vi "Configure Slave Test.vi"(8 "error in (no error)":errorcluster) -> (0 "error out":errorcluster)   [LabVIEW 2015]
uses:
  Tests/Controls/Test Config.ctl
  Tests/Controls/Gas Mixture.ctl
  CAN Communication/PAS/Typedefs/ADC Gains.ctl
  Tests/Controls/Filter Sequence.ctl
  Tests/Controls/Functional Test.ctl
  CAN Communication/PAS/PAS.lvclass
panel:
  in  "Test Config":T1={"Chopper RPM"=140, "IR Power"=5, "Conc Tolerance"=0.0, "Gas Stable Time"=0, "A-D Settle"=0, "Samples"=0, "Filter Time"=0, "Gas Mixtures"=[], "Filter Sequences"=[], "Functional Test"={"Mic Test ON ADC Max"=0.0, "Mic Test ON ADC Min"=0.0, "Mic Test OFF ADC Max"=0.0, "Mic Test OFF ADC Min"=0.0, "Mic Test IC ADC Max"=0.0, "Mic Test IC ADC Min"=0.0, "IR Emitter ON ADC Max"=0.0, "IR Emitter ON ADC Min"=0.0, "IR Emitter OFF ADC Max"=0.0, "IR Emitter OFF ADC Min"=0.0}, "Initial Flow Rate"=0.0, "Max Flow Rate"=0.0} {"Gas Mixtures"."ADC Gains" items=["0"=0, "3"=3, "4"=4, "5"=5, "6"=6, "7"=7]; "Conc Tolerance" min=0.0 max=100.0 step=1.0; "IR Power" min=2 max=5 step=1; "Chopper RPM" min=140 max=1000 step=1}
  in  "Remove Filter":bool
  in  "Max Flow Rate":sgl caption="Max Flow Rate (ccm)"
  in  "Initial Flow Rate":sgl caption="Initial Flow Rate (ccm)"
  in  "Down Button":bool
  in  "Up Button":bool
  in  "Edit Gas":bool
  in  "Add Gas":bool
  in  "Remove Gas":bool
  in  "Phase Per Filter":i32(listbox)=-2
  in  "Filter Time":u16 caption="Filter Settling Time (s)"
  in  "Samples":u16
  in  "A-D Settle":u16 caption="ADC Sampling Time (ms)"
  in  "Gas Stable Time":u16 caption="Gas Stability Time (s)"
  in  "Conc Tolerance":dbl caption="Concentration Tolerance (%)" min=0.0 max=100.0 step=1.0
  in  "IR Power":u8=5 caption="IR Power (W)" min=2 max=5 step=1
  in  "Chopper RPM":u16=140 caption="Chopper Frequency (RPM)" min=140 max=1000 step=1
  in  "Gas Mixtures":i32(listbox)=-2
  out "Cancelled?":bool
  in  "Cancel Button":bool
  in  "OK Button":bool
  out "Test Sequence":i32(listbox)=-2
  # "Configure Test"
  # "Hover over the controls\nto learn more about \nthe configuraton settings"
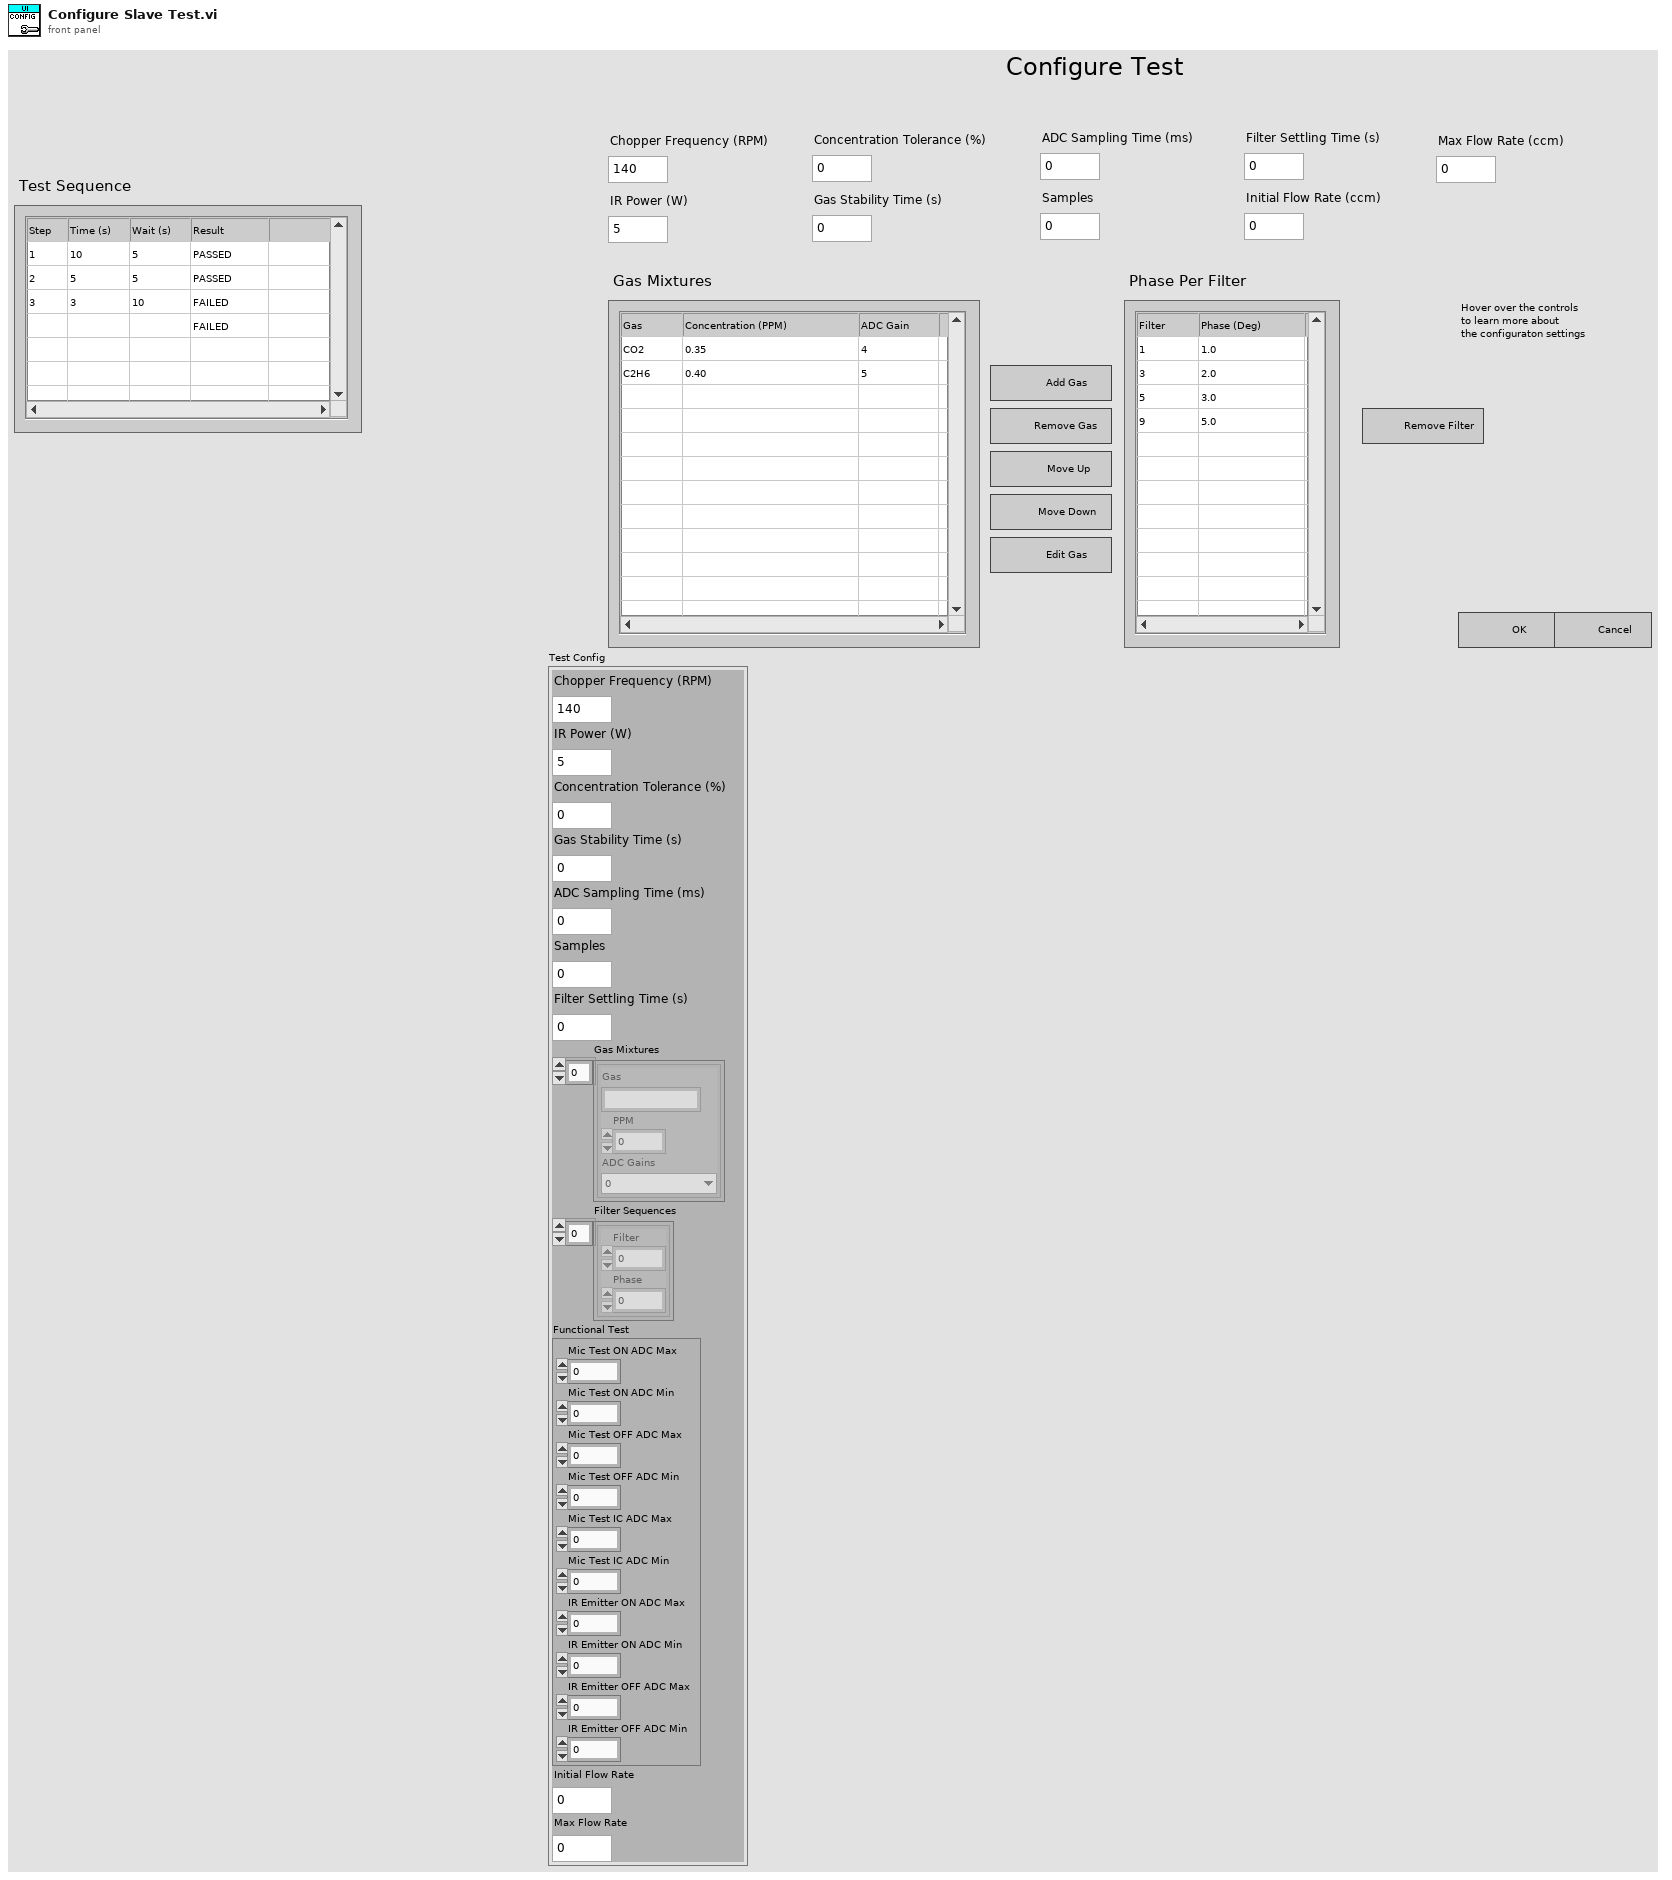
[diagram p1: front panel]
types:
  T1 = typedef "Test Config.ctl" = cluster{"Chopper RPM":u16, "IR Power":u8, "Conc Tolerance":dbl, "Gas Stable Time":u16, "A-D Settle":u16, "Samples":u16, "Filter Time":u16, "Gas Mixtures":T2[], "Filter Sequences":T4[], "Functional Test":T5, "Initial Flow Rate":sgl, "Max Flow Rate":sgl}
  T2 = typedef "Gas Mixture.ctl" = cluster{"Gas":string, "PPM":dbl, "ADC Gains":T3}
  T3 = typedef "PAS.lvclass/ADC Gains.ctl" = u16
  T4 = typedef "Filter Sequence.ctl" = cluster{"Filter":u8, "Phase":dbl}
  T5 = typedef "Functional Test.ctl" = cluster{"Mic Test ON ADC Max":dbl, "Mic Test ON ADC Min":dbl, "Mic Test OFF ADC Max":dbl, "Mic Test OFF ADC Min":dbl, "Mic Test IC ADC Max":dbl, "Mic Test IC ADC Min":dbl, "IR Emitter ON ADC Max":dbl, "IR Emitter ON ADC Min":dbl, "IR Emitter OFF ADC Max":dbl, "IR Emitter OFF ADC Min":dbl}
  T6 = typedef "LVPoint32TypeDef.ctl" = cluster{"Horizontal":i32, "Vertical":i32}
  T7 = typedef "LVRowAndColumnTypeDef.ctl" = cluster{"Row":i32, "Column":i32}
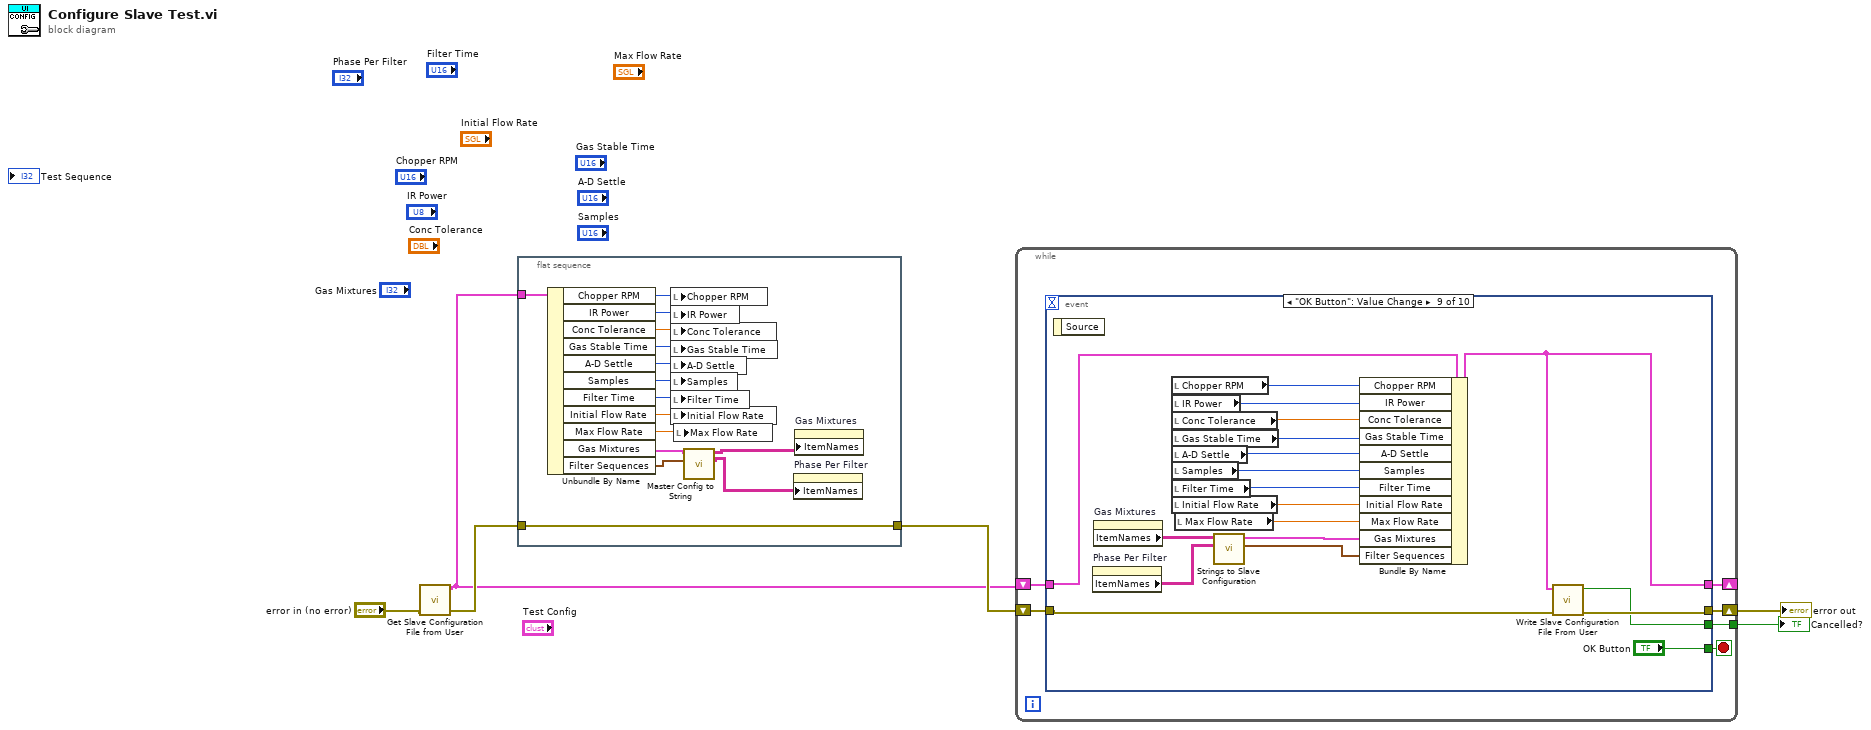
[diagram p0: block diagram]
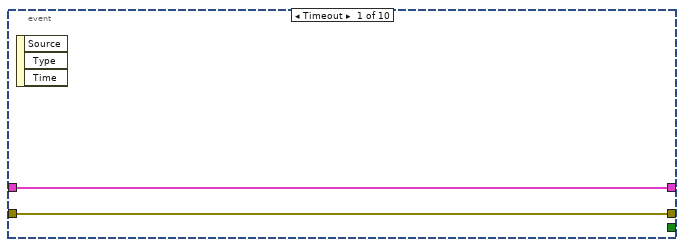
[diagram p2: hidden frame]
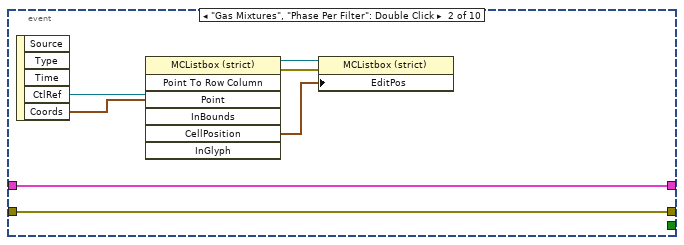
[diagram p3: hidden frame]
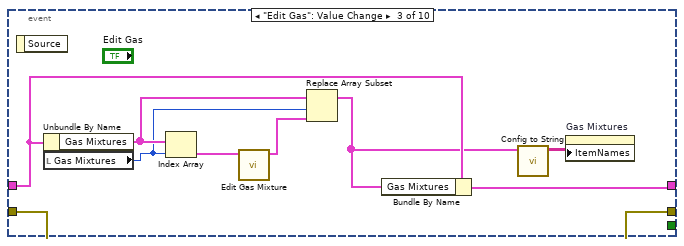
[diagram p4: hidden frame]
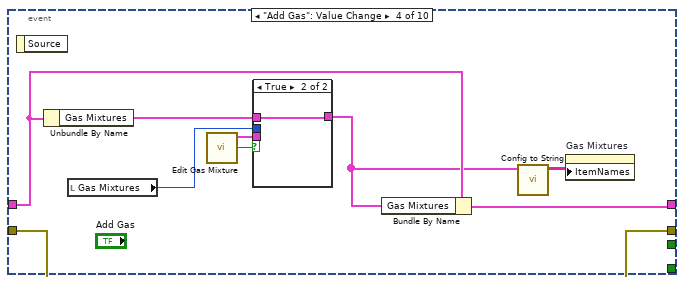
[diagram p5: hidden frame]
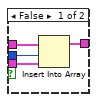
[diagram p6: hidden frame]
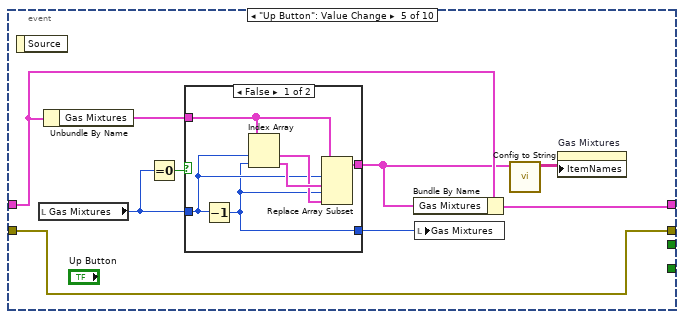
[diagram p7: hidden frame]
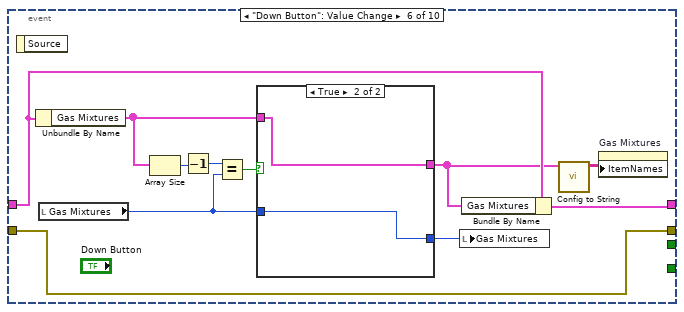
[diagram p9: hidden frame]
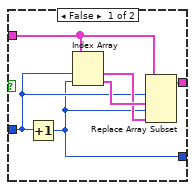
[diagram p10: hidden frame]
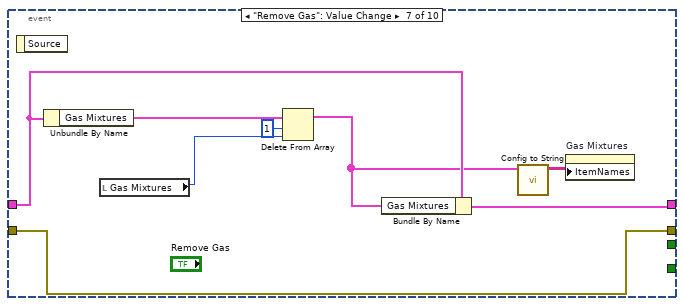
[diagram p11: hidden frame]
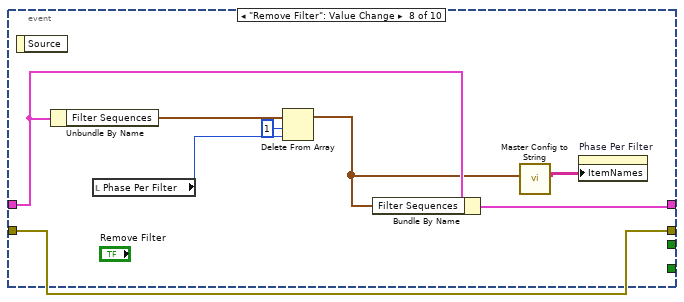
[diagram p12: hidden frame]
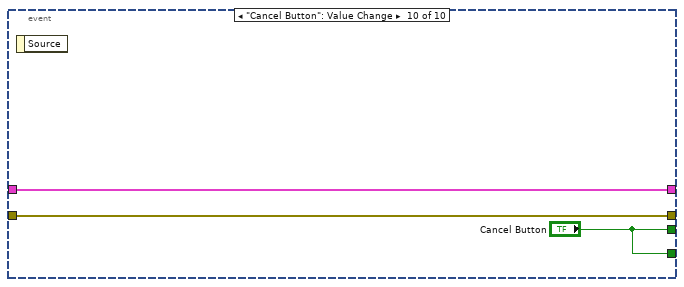
[diagram p13: hidden frame]
diagram:
  n1 = call "Get Slave Configuration File from User.vi"("error in"="error in (no error)") -> ("error out"=w2:errorcluster, "Test Config"=w1:T1)  [unwired: 7 in, 2 out]
  n2 = flat-sequence {
    tunnel: w1 -> [w20]
    tunnel: w2 -> [w21]
    tunnel: [w21] -> w4
    frame #0 {
      n3 = Unbundle By Name(w20) -> ("Chopper RPM"=w19:u16, "IR Power"=w18:u8, "Conc Tolerance"=w17:dbl, "Gas Stable Time"=w16:u16, "A-D Settle"=w15:u16, "Samples"=w14:u16, "Filter Time"=w13:u16, "Initial Flow Rate"=w12:sgl, "Max Flow Rate"=w11:sgl, "Gas Mixtures"=w10:T2[], "Filter Sequences"=w9:T4[])
      n4 = local write "Chopper RPM"(w19) -> ()
      n5 = local write "IR Power"(w18) -> ()
      n6 = local write "Conc Tolerance"(w17) -> ()
      n7 = local write "Gas Stable Time"(w16) -> ()
      n8 = local write "A-D Settle"(w15) -> ()
      n9 = local write "Samples"(w14) -> ()
      n10 = local write "Filter Time"(w13) -> ()
      n11 = local write "Initial Flow Rate"(w12) -> ()
      n12 = local write "Max Flow Rate"(w11) -> ()
      n13 = call "Master Config to String.vi"("Filter Sequences"=w9, "Gas Mixtures"=w10) -> ("Filter"=w7:string[][], "Gas"=w8:string[][])  [unwired: 8 in]
      n14 = property on="Phase Per Filter" class="MCListbox (strict)"("ItemNames"=w7) -> ()  [unwired: 2 in, 2 out]
      n15 = property on="Gas Mixtures" class="MCListbox (strict)"("ItemNames"=w8) -> ()  [unwired: 2 in, 2 out]
    }
  }
  n16 = while {
    tunnel: [w27] -> w6
    shift-right: [w24] -> w5
    shift-left: w4 -> [w25]
    shift-right: [w22] -> _
    shift-left: w1 -> [w23]
    stop <- w26 stop-if-true
    n17 = event shown="[8] \"OK Button\": Value Change" {
      selector: _ -> [_ _ _ _ _ _ _ _ _ _]
      dyn-events: _ -> [_ _ _ _ _ _ _ _ _ _]
      timeout: _ -> [_ _ _ _ _ _ _ _ _ _]
      tunnel: [_ _ _ _ _ _ _ _ w125 "Cancel Button"] -> w27
      tunnel: [_ _ _ _ _ _ _ _ "OK Button" "Cancel Button"] -> w26
      tunnel: w25 -> [w29 w31 w44 w54 w68 w87 w103 w111 w127 w132]
      tunnel: [w29 w31 w44 w54 w68 w87 w103 w111 w129 w132] -> w24
      tunnel: w23 -> [w28 w30 w40 w52 w67 w86 w102 w110 w126 w131]
      tunnel: [w28 w30 w39 w51 w66 w85 w101 w109 w121 w131] -> w22
      event Timeout {
        n18 = event-data() -> ()  [unwired: 1 in, 3 out]
      }
      event "Gas Mixtures", "Phase Per Filter": Double Click {
        n19 = event-data() -> ("CtlRef"=w36:refnum<vi>, "Coords"=w35:T6)  [unwired: 1 in, 3 out]
        n20 = invoke class="MCListbox (strict)" method="Point To Row Column"(reference=w36, "Point"=w35) -> (reference out=w34:refnum<vi>, error out=w33:errorcluster, "CellPosition"=w32:T7)  [unwired: 5 in, 4 out]
        n21 = property class="MCListbox (strict)"(reference=w34, error in=w33, "EditPos"=w32) -> ()  [unwired: 2 out]
      }
      event "Edit Gas": Value Change {
        n22 = event-data() -> ()  [unwired: 1 in, 1 out]
        n23 = Unbundle By Name(w40) -> ("Gas Mixtures"=w43:T2[])
        n24 = local read "Gas Mixtures"() -> (w42:i32)
        n25 = Index Array(array=w43, index=w42) -> (element=w45:T2)
        n26 = call "Edit Gas Mixture.vi"("Gas Mixture In"=w45) -> ("Gas Mixture Out"=w41:T2)  [unwired: 8 in, 2 out]
        n27 = Replace Array Subset(array=w43, new element=w41, index=w42) -> (w38:T2[])
        n28 = Bundle By Name(cluster=w40, "Gas Mixtures"=w38) -> (w39:T1)
        n29 = call "Config to String.vi"("Gas Sequence"=w38) -> ("Gas"=w37:string[][])  [unwired: 10 in]
        n30 = property on="Gas Mixtures" class="MCListbox (strict)"("ItemNames"=w37) -> ()  [unwired: 2 in, 2 out]
      }
      event "Add Gas": Value Change {
        n31 = event-data() -> ()  [unwired: 1 in, 1 out]
        n32 = Unbundle By Name(w52) -> ("Gas Mixtures"=w48:T2[])
        n33 = local read "Gas Mixtures"() -> (w46:i32)
        n34 = call "Edit Gas Mixture.vi"() -> ("Cancel?"=w47:bool, "Gas Mixture Out"=w53:T2)  [unwired: 9 in, 1 out]
        n35 = case shown="True" w47 {
          tunnel: w46 -> [w58 _]
          tunnel: w53 -> [w57 _]
          tunnel: [w56 w59] -> w50
          tunnel: w48 -> [w55 w59]
          frame False {
            n36 = Insert Into Array(array=w55, index=w58, new element=w57) -> (w56:T2[])
          }
          frame True {
          }
        }
        n37 = Bundle By Name(cluster=w52, "Gas Mixtures"=w50) -> (w51:T1)
        n38 = call "Config to String.vi"("Gas Sequence"=w50) -> ("Gas"=w49:string[][])  [unwired: 10 in]
        n39 = property on="Gas Mixtures" class="MCListbox (strict)"("ItemNames"=w49) -> ()  [unwired: 2 in, 2 out]
      }
      event "Up Button": Value Change {
        n40 = event-data() -> ()  [unwired: 1 in, 1 out]
        n41 = local read "Gas Mixtures"() -> (w62:i32)
        n42 = Unbundle By Name(w67) -> ("Gas Mixtures"=w64:T2[])
        n43 = Equal To 0?(x=w62) -> (x = 0?=w61:bool)
        n44 = case shown="False" w61 {
          tunnel: w64 -> [w74 w76]
          tunnel: [w71 w76] -> w63
          tunnel: w62 -> [w70 w75]
          tunnel: [w69 w75] -> w60
          frame False {
            n45 = Decrement(x=w70) -> (x-1=w69:i32)
            n46 = Index Array(array=w74, index #1=w70, index #2=w69) -> (element #1=w72:T2, element #2=w73:T2)
            n47 = Replace Array Subset(array=w74, new element #1=w73, index #1=w70, new element #2=w72, index #2=w69) -> (w71:T2[])
          }
          frame True {
          }
        }
        n48 = Bundle By Name(cluster=w67, "Gas Mixtures"=w63) -> (w66:T1)
        n49 = local write "Gas Mixtures"(w60) -> ()
        n50 = call "Config to String.vi"("Gas Sequence"=w63) -> ("Gas"=w65:string[][])  [unwired: 10 in]
        n51 = property on="Gas Mixtures" class="MCListbox (strict)"("ItemNames"=w65) -> ()  [unwired: 2 in, 2 out]
      }
      event "Down Button": Value Change {
        n52 = event-data() -> ()  [unwired: 1 in, 1 out]
        n53 = Unbundle By Name(w86) -> ("Gas Mixtures"=w82:T2[])
        n54 = local read "Gas Mixtures"() -> (w79:i32)
        n55 = Array Size(array=w82) -> (size(s)=w81:i32)
        n56 = Decrement(x=w81) -> (x-1=w80:i32)
        n57 = Equal?(x=w80, y=w79) -> (x = y?=w78:bool)
        n58 = case shown="True" w78 {
          tunnel: w82 -> [w93 w95]
          tunnel: [w90 w95] -> w83
          tunnel: w79 -> [w89 w94]
          tunnel: [w88 w94] -> w77
          frame False {
            n59 = Increment(x=w89) -> (x+1=w88:i32)
            n60 = Index Array(array=w93, index #1=w89, index #2=w88) -> (element #1=w91:T2, element #2=w92:T2)
            n61 = Replace Array Subset(array=w93, new element #1=w92, index #1=w89, new element #2=w91, index #2=w88) -> (w90:T2[])
          }
          frame True {
          }
        }
        n62 = local write "Gas Mixtures"(w77) -> ()
        n63 = Bundle By Name(cluster=w86, "Gas Mixtures"=w83) -> (w85:T1)
        n64 = call "Config to String.vi"("Gas Sequence"=w83) -> ("Gas"=w84:string[][])  [unwired: 10 in]
        n65 = property on="Gas Mixtures" class="MCListbox (strict)"("ItemNames"=w84) -> ()  [unwired: 2 in, 2 out]
      }
      event "Remove Gas": Value Change {
        n66 = event-data() -> ()  [unwired: 1 in, 1 out]
        n67 = Unbundle By Name(w102) -> ("Gas Mixtures"=w98:T2[])
        n68 = local read "Gas Mixtures"() -> (w97:i32)
        n69 = Delete From Array(array=w98, length=1, index=w97) -> (array with subset deleted=w100:T2[])  [unwired: 1 out]
        n70 = Bundle By Name(cluster=w102, "Gas Mixtures"=w100) -> (w101:T1)
        n71 = call "Config to String.vi"("Gas Sequence"=w100) -> ("Gas"=w99:string[][])  [unwired: 10 in]
        n72 = property on="Gas Mixtures" class="MCListbox (strict)"("ItemNames"=w99) -> ()  [unwired: 2 in, 2 out]
      }
      event "Remove Filter": Value Change {
        n73 = event-data() -> ()  [unwired: 1 in, 1 out]
        n74 = Unbundle By Name(w110) -> ("Filter Sequences"=w108:T4[])
        n75 = local read "Phase Per Filter"() -> (w107:i32)
        n76 = Delete From Array(array=w108, length=1, index=w107) -> (array with subset deleted=w105:T4[])  [unwired: 1 out]
        n77 = Bundle By Name(cluster=w110, "Filter Sequences"=w105) -> (w109:T1)
        n78 = call "Master Config to String.vi"("Filter Sequences"=w105) -> ("Filter"=w104:string[][])  [unwired: 9 in, 1 out]
        n79 = property on="Phase Per Filter" class="MCListbox (strict)"("ItemNames"=w104) -> ()  [unwired: 2 in, 2 out]
      }
      event "OK Button": Value Change {
        n80 = event-data() -> ()  [unwired: 1 in, 1 out]
        n81 = property on="Phase Per Filter" class="MCListbox (strict)"() -> ("ItemNames"=w124:string[][])  [unwired: 2 in, 2 out]
        n82 = property on="Gas Mixtures" class="MCListbox (strict)"() -> ("ItemNames"=w128:string[][])  [unwired: 2 in, 2 out]
        n83 = local read "Chopper RPM"() -> (w120:u16)
        n84 = local read "IR Power"() -> (w119:u8)
        n85 = local read "Conc Tolerance"() -> (w118:dbl)
        n86 = local read "Gas Stable Time"() -> (w117:u16)
        n87 = local read "A-D Settle"() -> (w116:u16)
        n88 = local read "Samples"() -> (w115:u16)
        n89 = local read "Filter Time"() -> (w114:u16)
        n90 = local read "Initial Flow Rate"() -> (w113:sgl)
        n91 = local read "Max Flow Rate"() -> (w112:sgl)
        n92 = call "Strings to Slave Configuration.vi"("Filter"=w124, "Gas"=w128) -> ("Filter Sequences Out"=w122:T4[], "Gas Mixtures Out"=w123:T2[])  [unwired: 8 in]
        n93 = Bundle By Name(cluster=w126, "Chopper RPM"=w120, "IR Power"=w119, "Conc Tolerance"=w118, "Gas Stable Time"=w117, "A-D Settle"=w116, "Samples"=w115, "Filter Time"=w114, "Initial Flow Rate"=w113, "Max Flow Rate"=w112, "Gas Mixtures"=w123, "Filter Sequences"=w122) -> (w121:T1)
        n94 = call "Write Slave Configuration File From User.vi"("error in"=w127, "Test Config"=w121) -> ("error out"=w129:errorcluster, "Cancelled?"=w125:bool)  [unwired: 8 in]
      }
      event "Cancel Button": Value Change {
        n95 = event-data() -> ()  [unwired: 1 in, 1 out]
      }
    }
  }
  "error out" <- w5
  "Cancelled?" <- w6
